vi "Test Prepare Path Returns Unique File Name if Existing Given.vi"(11 "Test Case In":refnum<class "Report Plugin Test.lvclass">) -> (0 "error out":errorcluster, 3 "Test Case Out":refnum<class "Report Plugin Test.lvclass">)   [LabVIEW 2020, in "Report Plugin Test.lvclass"]
uses:
  Report Plugin Test.lvclass
  C:/git/astemes-lunit/source/Framework/Report Plugin/Report Plugin.lvclass
  C:/Program Files (x86)/National Instruments/LabVIEW 2020/vi.lib/Astemes/LUnit/Test Case.lvclass
  <vilib>/Astemes/LUnit/Test Case.lvclass/Test Case.ctl
  <vilib>/Astemes/LUnit/Core/LUnit Test Case/Private/Append Pass Result.vi
  <vilib>/Astemes/LUnit/Core/LUnit Test Case/Private/Append Fail Result.vi
  e1eeebb6-1c69-40ac-a018-3a09ac31808e.vi/9c5d11cd-9439-4240-a1ee-d9baace9c924.vi
  <vilib>/Astemes/LUnit/Core/LUnit Test Case/Private/Run In UI.vi
  <vilib>/Utility/error.llb/Clear Errors.vi
  Report Plugin Test.lvclass/Report Plugin Test.ctl
  source/Framework/Report Plugin/Report Plugin.lvclass
  C:/git/astemes-lunit/source/Framework/Plugin/Plugin.lvclass
  C:/Program Files (x86)/National Instruments/LabVIEW 2020/vi.lib/Astemes/LUnit/LUnit Runnable.lvclass
  C:/git/astemes-lunit/tests/Report Plugin Test/Report Plugin Test.lvclass
  <vilib>/Astemes/LUnit/Palette/Advanced Assertions/LUnit Advanced Assertions.lvlib
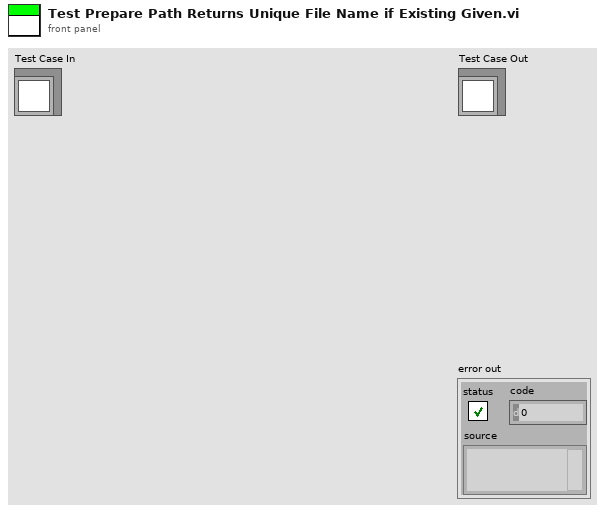
[diagram p1: front panel]
types:
  T1 = enum16{"open", "replace", "create", "open or create", "replace or create", "replace or create with confirmation"}
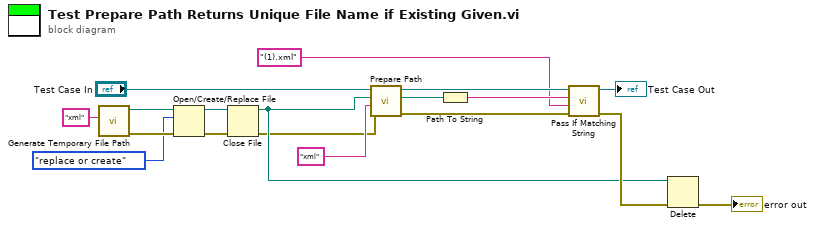
[diagram p0: block diagram]
diagram:
  n1 = call <vilib>:"Generate Temporary File Path.vi"("Temporary File Extension (tmp)"="xml") -> ("error out"=w7:errorcluster, "Unique Temporary File Path"=w8:path)  [unwired: 9 in]
  n2 = Open/Create/Replace File(file path (use dialog)=w8, error in=w7, operation (0:open)=T1."replace or create") -> (refnum out=w11:refnum<file>, error out=w10:errorcluster)  [unwired: 3 in, 1 out]
  n3 = Close File(refnum=w11, error in=w10) -> (path=w5:path, error out=w4:errorcluster)
  n4 = call "Prepare Path.vi"("error in (no error)"=w4, "Extenssion"="xml", "File Path in"=w5, "Plugin In"="Test Case In") -> ("error out"=w14:errorcluster, "Modified Path"=w13:path, "Plugin Out"=w15:refnum<class "Report Plugin Test.lvclass">)  [unwired: 5 in]
  n5 = Path To String(path=w13) -> (string=w2:string)
  n6 = call <vilib>:"Pass If Matching String.vi"("error in (no error)"=w14, "Regular Expression"="(1).xml" ("File Path in"), "String"=w2, "LUnit Test Case In"=w15) -> ("error out"=w17:errorcluster, "LUnit Test Case Out"=→"Test Case Out":refnum<class "Report Plugin Test.lvclass">)  [unwired: 6 in]
  n7 = Delete(path (use dialog)=w5, error in=w17) -> (error out=→"error out":errorcluster)  [unwired: 3 in, 2 out]
